vi "Robcomm_Run.vi"(2 "Program name":string="LDP1", 3 "DDE Service name":string="ROBCOMM") -> (1 "Error?":bool)   [LabVIEW 2012]
panel:
  out "Command":string="RUN"
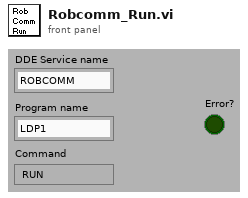
[diagram p1: front panel]
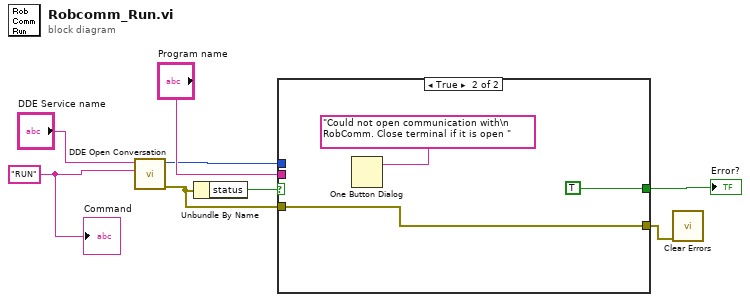
[diagram p0: block diagram]
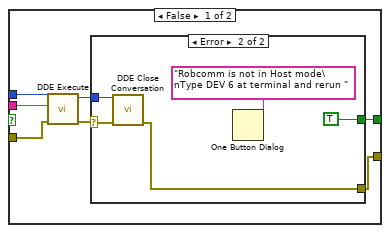
[diagram p2: hidden frame]
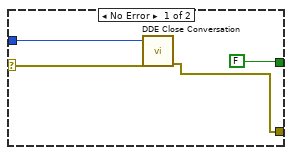
[diagram p3: hidden frame]
diagram:
  w3 = "RUN" ("topic")
  n1 = call <vilib>:"DDE Open Conversation.vi"("topic"=w3, "service"="DDE Service name") -> ("error out"=w7:errorcluster, "conversation refnum"=w4:u32)  [unwired: 6 in]
  n2 = Unbundle By Name(w7) -> ("status"=w6:bool)
  n3 = case shown="True" w6 {
    tunnel: w4 -> [w15 _]
    tunnel: "Program name" -> [w13 _]
    tunnel: w7 -> [w11 w26]
    tunnel: [w10 TRUE] -> w2
    tunnel: [w9 w26] -> w1
    frame False {
      n4 = call <vilib>:"DDE Execute.vi"("error in (no error)"=w11, "command"=w13, "conversation refnum in"=w15) -> ("error out"=w12:errorcluster, "conversation refnum out"=w14:u32)  [unwired: 5 in]
      n5 = case shown="Error" w12 {
        selector: w12 -> [w18 w24]
        tunnel: w14 -> [w19 w23]
        tunnel: [FALSE TRUE] -> w10
        tunnel: [w16 w22] -> w9
        frame No Error {
          n6 = call <vilib>:"DDE Close Conversation.vi"("error in (no error)"=w18, "conversation refnum"=w19) -> ("error out"=w16:errorcluster)  [unwired: 7 in]
        }
        frame Error {
          n7 = call <vilib>:"DDE Close Conversation.vi"("error in (no error)"=w24, "conversation refnum"=w23) -> ("error out"=w22:errorcluster)  [unwired: 7 in]
          n8 = One Button Dialog(message="Robcomm is not in Host mode\nType DEV 6 at terminal and rerun ") -> ()  [unwired: 1 in, 1 out]
        }
      }
    }
    frame True {
      n9 = One Button Dialog(message="Could not open communication with\n RobComm. Close terminal if it is open ") -> ()  [unwired: 1 in, 1 out]
    }
  }
  "Error?" <- w2
  n10 = call <vilib>:"Clear Errors.vi"("error in (no error)"=w1) -> ()  [unwired: 6 in, 1 out]
  "Command" <- w3
